vi "FPGA Check (RT).vi"() -> ()   [LabVIEW 2019]
uses:
  <vilib>/rvi/interface/nirviOpenFPGA/nirviOpenFPGA.xnode
  <vilib>/rvi/interface/nirviMethod/nirviMethod.xnode
  <vilib>/rvi/interface/nirviReadWriteControl/nirviReadWriteControl.xnode
  FPGA Bitfiles/LSDurabilityMain_Alternate_Two.lvbitx
  <vilib>/FPGAPlugInAG/sbRIO-9626/niLvFpga_Open_sbRIO-9626.vi
  <vilib>/FPGAPlugInAG/sbRIO-9626/niLvFpga_Reset_sbRIO-9626.vi
  <vilib>/FPGAPlugInAG/sbRIO-9626/niLvFpga_Run_sbRIO-9626.vi
  <vilib>/rvi/errors/niLvFpgaMergeErrorWithErrorCode.vi
  <vilib>/rvi/errors/niLvFpgaAdjustHostInterfaceError.vi
panel:
  in  "pause":bool
  out "Opens Detected":i16[](array[numeric])
  in  "Duty (Ticks)":i32=1613760
  in  "PWM Period (Ticks)":u32=1640000
  out "Bank1On":bool
  out "Bank1Active":bool
  out "Waveform Chart 2":cluster{dbl, i16, i16}(graph)
  out "AI Loop Time (usec)":u32
  in  "Bank1Const(On/Off)":bool
  in  "Bank1(Pulse/Const)":bool
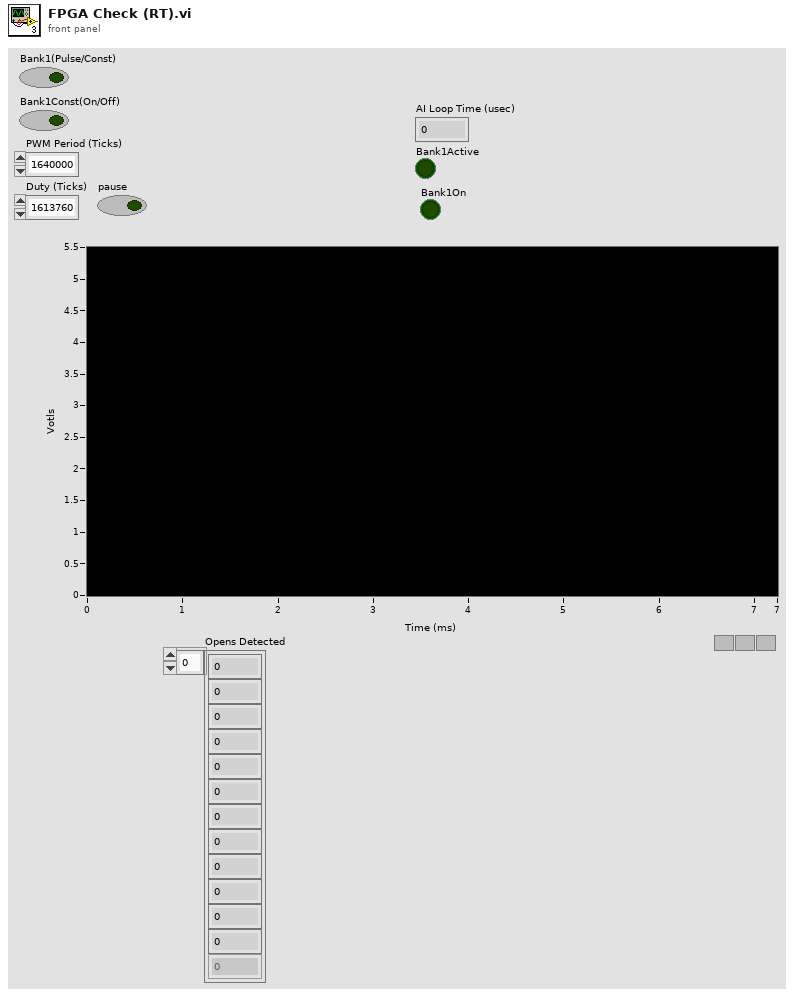
[diagram p1: front panel]
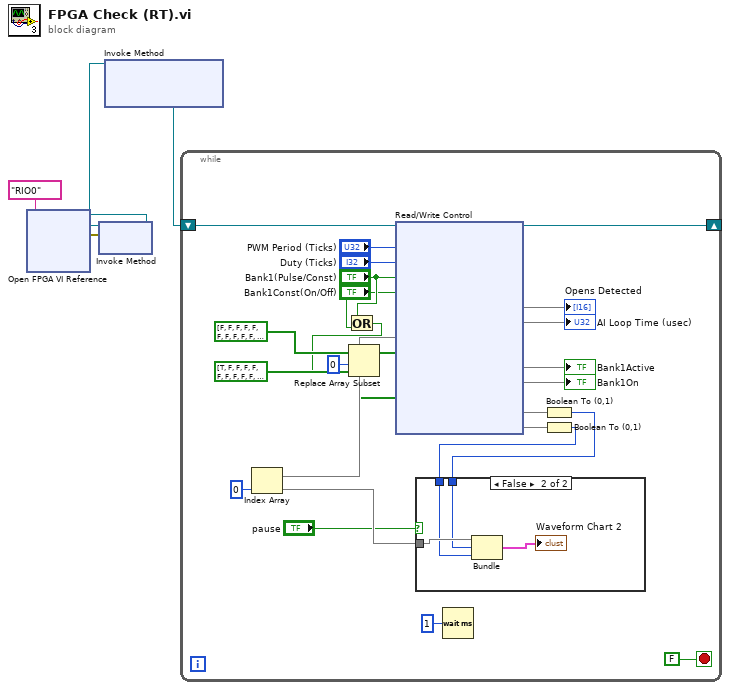
[diagram p0: block diagram]
diagram:
  n1 = xnode "Open FPGA VI Reference"("resource name"=tag "RIO0") -> ("FPGA VI Reference Out"=w4:refnum<k20>, "error out"=w5:errorcluster)  [unwired: 1 in]
  n2 = xnode "Invoke Method"("FPGA VI Reference In"=w4, "error in"=w5) -> ("FPGA VI Reference Out"=w2:refnum<k20>)  [unwired: 1 out]
  n3 = xnode "Invoke Method"("FPGA VI Reference In"=w2) -> ("FPGA VI Reference Out"=w1:refnum<k20>)  [unwired: 2 in, 1 out]
  n4 = while {
    shift-right: [w28] -> _
    shift-left: w1 -> [w29]
    stop <- FALSE stop-if-true
    n5 = Or(x="Bank1(Pulse/Const)", y="Bank1Const(On/Off)") -> (x .or. y?=w11:bool)
    n6 = Replace Array Subset(array=bool[] [FALSE, FALSE, FALSE, FALSE, FALSE, FALSE, FALSE, FALSE, FALSE, FALSE, FALSE, FALSE] ("Enable Opens"), new element=w11, index=0) -> (w15:bool[])
    n7 = xnode "Read/Write Control"("FPGA VI Reference In"=w29, "PWM Period (Ticks)"="PWM Period (Ticks)", "Duty (Ticks)"="Duty (Ticks)", "Bank1(Pulse/Const)"="Bank1(Pulse/Const)", "Bank1Const(On/Off)"="Bank1Const(On/Off)", "Enable Opens"=w15, "Enable Readings"=bool[] [TRUE, FALSE, FALSE, FALSE, FALSE, FALSE, FALSE, FALSE, FALSE, FALSE, FALSE, FALSE] ("Enable Opens")) -> ("FPGA VI Reference Out"=w28:refnum<k20>, "Opens Detected"=→"Opens Detected", "AI Loop Time (usec)"=→"AI Loop Time (usec)", "Analog Inputs"=w24, "Bank1Active"=→"Bank1Active", "Bank1On"=→"Bank1On", "Open"=w9, "Bankvalid"=w8)  [unwired: 1 in, 1 out]
    n8 = Index Array(array=w24, index=0) -> (element=w22)
    n9 = Wait (ms)(milliseconds to wait=u32 1) -> ()  [unwired: 1 out]
    n10 = Boolean To (0,1)(Boolean=w9) -> (0, 1=w7:i16)
    n11 = Boolean To (0,1)(Boolean=w8) -> (0, 1=w6:i16)
    n12 = case shown="False" "pause" {
      tunnel: w22 -> [_ w34]
      tunnel: w7 -> [_ w32]
      tunnel: w6 -> [_ w31]
      frame True {
      }
      frame False {
        n13 = Bundle(w34, w32, w31) -> (→"Waveform Chart 2":cluster{void, i16, i16})  [unwired: 1 in]
      }
    }
  }
